vi "New Valve.vi"(8 "error in (no error)":errorcluster, 11 "valve color":T1) -> (0 "error out":errorcluster, 3 "Valve Item out":refnum<class "Valve Item.lvclass">)   [LabVIEW 2020, in "BetterDragAndDropDemo.lvlib" / "Valve Item.lvclass"]
uses:
  Valve Item.lvclass
  valve color.ctl
  Valve Item.lvclass/Valve Item.ctl
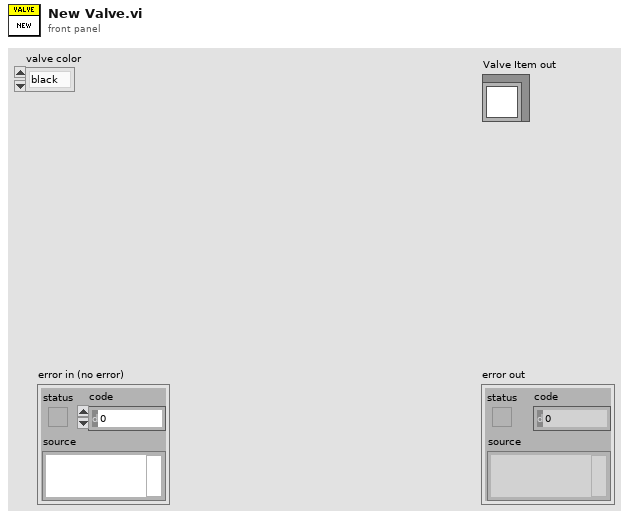
[diagram p1: front panel]
types:
  T1 = typedef "BetterDragAndDropDemo.lvlib/Valve Item.lvclass/valve color.ctl" = enum16{"black", "red"}
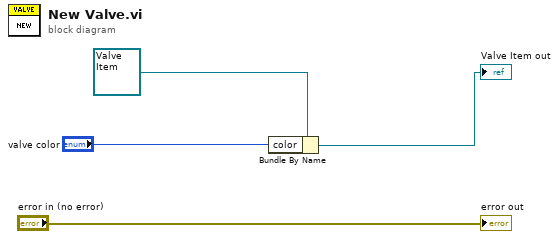
[diagram p0: block diagram]
diagram:
  n1 = Bundle By Name(cluster=refnum<class "Valve Item.lvclass"> refnum ("Valve Item out"), "color"="valve color") -> (→"Valve Item out":refnum<class "Valve Item.lvclass">)
  "error out" <- "error in (no error)"
